vi "_f_bronkhorstWriteAuto.vi"(6 "Delay Time (s)":dbl=0.4, 8 "error in (no error)":errorcluster, 11 "Datos":T1 caption="Nuevos valores" {"Ctrl01" format="%.1f"; "Ctrl03" format="%.1f"; "Ctrl02" format="%.1f"; "Ctrl04" format="%.1f"}) -> (0 "error out":errorcluster, 1 "Dispositivos":T2=[["3", "NO", "M0000013", "Air", "1", "ln/mn", "0", "0"], ["4", "NO", "M0000014", "Air", "1", "ln/mn", "0", "0"], ["5", "NO", "M0000015", "Air", "1", "ln/mn", "0", "0"], ["6", "NO", "M0000016", "Air", "1", "ln/mn", "0", "0"], ["7", "NO", "M0000017", "Air", "1", "ln/mn", "0", "0"], ["8", "NO", "M0000018", "Air", "1", "ln/mn", "0", "0"], ["9", "NO", "M0000019", "Air", "1", "ln/mn", "0", "0"], ["10", "NO", "M0000020", "Air", "1", "ln/mn", "0", "0"], ["11", "NO", "M0000021", "Air", "1", "ln/mn", "0", "0"]] caption="MassFlowControllers")   [LabVIEW 2013]
uses:
  _f_TablaBronkhorst.ctl
  Controles/P2018 Flujos Data.ctl
  _f_BronkhorstModuleControl.ctl
  P2022 TB INCAR GLOBALES.vi
panel:
  out "Nodo":i32
  out "Dispositivos 2":string[][](table)=[["3", "NO", "M0000013", "Air", "1", "ln/mn", "0", "0"], ["4", "NO", "M0000014", "Air", "1", "ln/mn", "0", "0"], ["5", "NO", "M0000015", "Air", "1", "ln/mn", "0", "0"], ["6", "NO", "M0000016", "Air", "1", "ln/mn", "0", "0"], ["7", "NO", "M0000017", "Air", "1", "ln/mn", "0", "0"], ["8", "NO", "M0000018", "Air", "1", "ln/mn", "0", "0"], ["9", "NO", "M0000019", "Air", "1", "ln/mn", "0", "0"], ["10", "NO", "M0000020", "Air", "1", "ln/mn", "0", "0"], ["11", "NO", "M0000021", "Air", "1", "ln/mn", "0", "0"]] caption="Nuevos valores"
  out "Enable(T)":bool=TRUE
  out "VISA Bronkhorst":refnum<visa-resource-name>
  out "Num. of nodes":u32=6
  # "Cambio de setpoints automático: espere........."
  # "4"
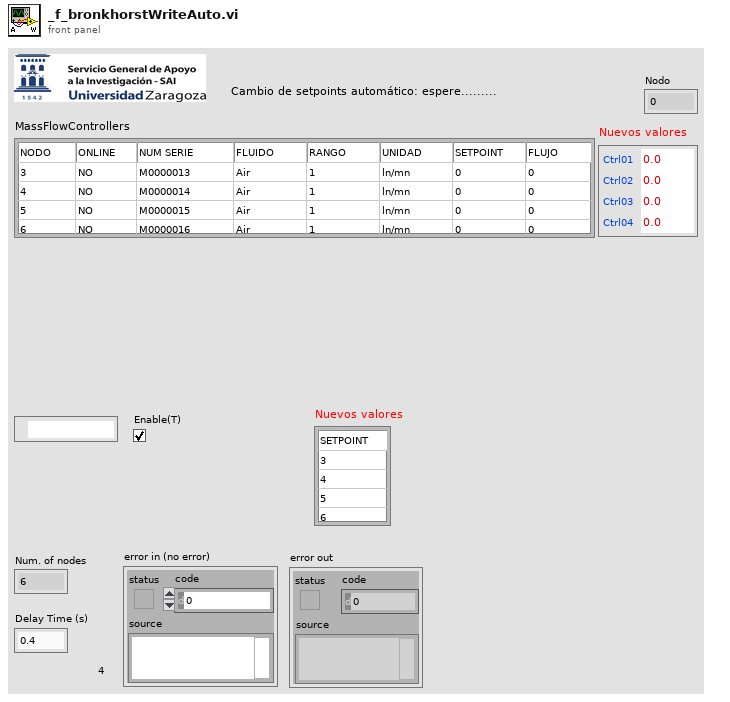
[diagram p1: front panel]
types:
  T1 = typedef "P2018 Flujos Data.ctl" = cluster{"Ctrl01":dbl, "Ctrl02":dbl, "Ctrl03":dbl, "Ctrl04":dbl}
  T2 = typedef "_f_TablaBronkhorst.ctl" = string[][]
  T3 = typedef "P2018 Bronkhorst Control.ctl" = cluster{"Dispositivos":T4, "NuevosSP":string[][], "Nodes":u32, "Delay(s)":dbl}
  T4 = typedef "_s_TablaBronkhorst.ctl" = string[][]
  T5 = typedef "P2018 Com Control.ctl" = cluster{"Flujo_1":refnum<visa-resource-name>, "Brk1":bool, "Flujo_2":refnum<visa-resource-name>, "Brk2":bool, "Flujo_3":refnum<visa-resource-name>, "Brk3":bool, "Flujo_4":refnum<visa-resource-name>, "Brk4":bool, "Eurothe":refnum<visa-resource-name>, "Eurot":bool, "Balanza":refnum<visa-resource-name>, "Bal":bool, "eValPos":refnum<visa-resource-name>, "eVal":bool, "flowbus":refnum<visa-resource-name>, "fb":bool}
  T6 = typedef "_f_BronkhorstModuleControl.ctl" = enum16{"RcharSerialNum", "RcharIdnString", "WuintFluidNum", "RuintFluidNum", "RcharFluidName", "RuintSensorType", "RfloatCap0", "RfloatCap100", "RcharCapUnitStr", "W%Setpoint", "R%Setpoint", "R%Measure", "WfloatSetpoint", "RfloatSetpoint", "RfloatMeasure ", "RfloatDensity", "WuintControlMode", "WcharRESET", "RfloatCounter", "RcharCounterUnit", "WfloatCounterLimit", "RfloatCounterLimit", "WcharCounterMode", "RcharCounterMode", "WcharCounterSPMode", "RcharCounterSPMode", "WcharCounterNewSP", "RcharCounterNewSP"}
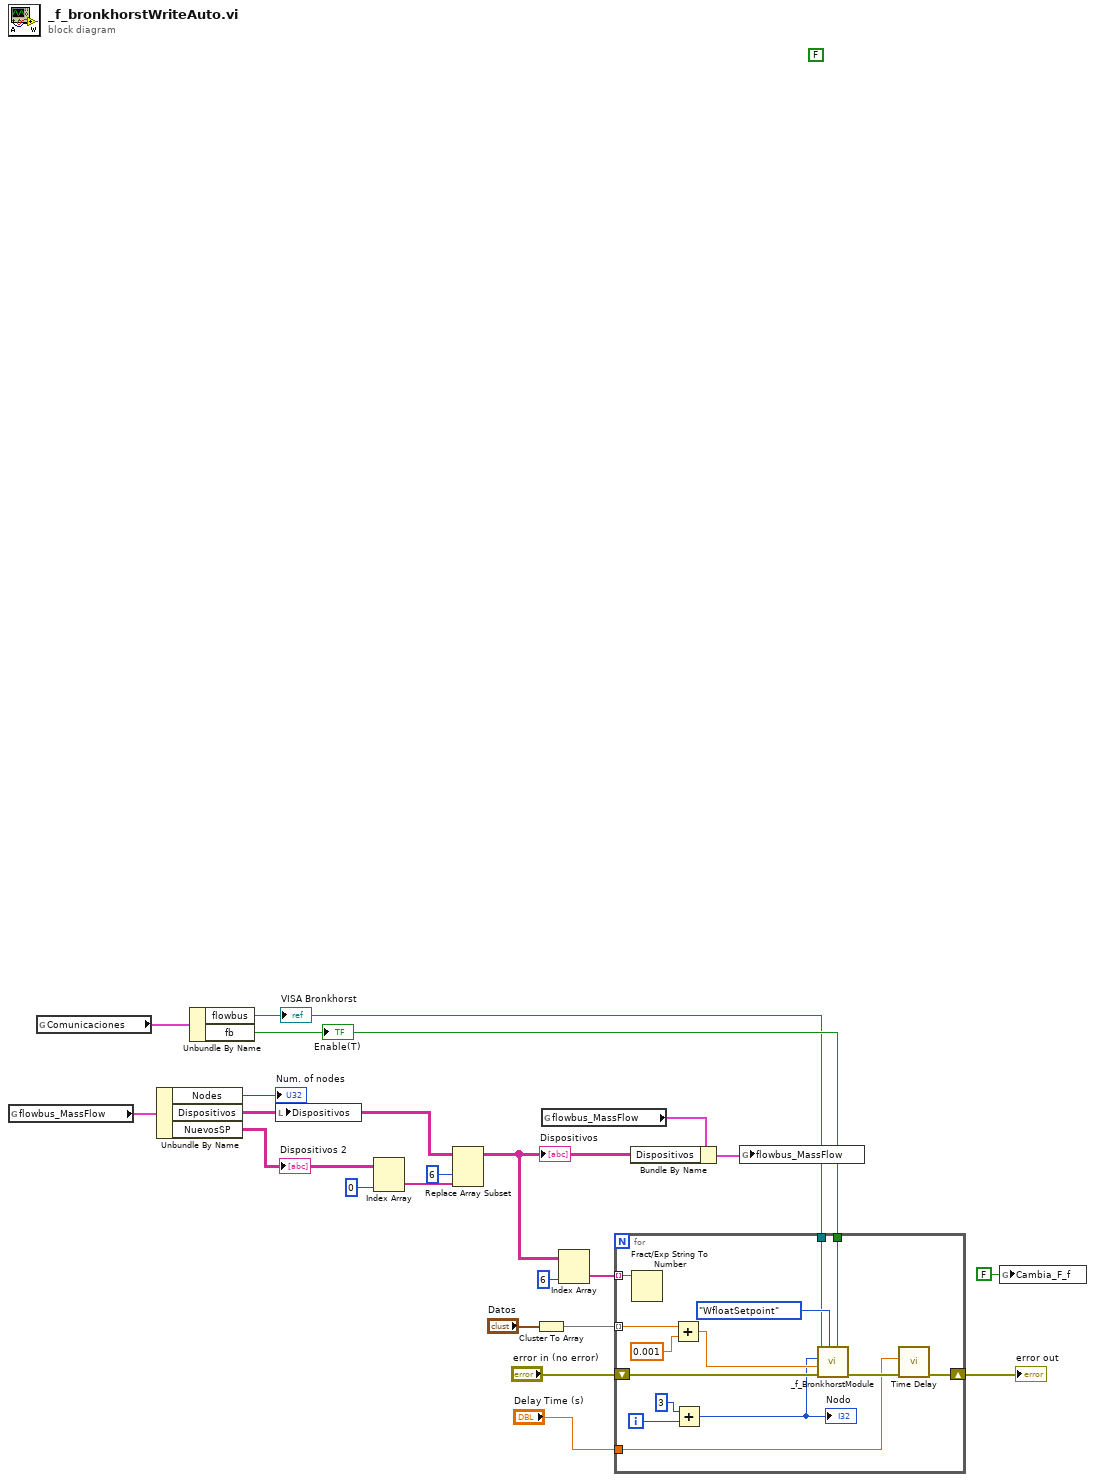
[diagram p0: block diagram]
diagram:
  (unwired) FALSE
  n1 = global read "P2022 TB INCAR GLOBALES.vi" "flowbus_MassFlow"() -> (w17:T3)
  n2 = global read "P2022 TB INCAR GLOBALES.vi" "Comunicaciones"() -> (w21:T5)
  n3 = Unbundle By Name(w17) -> ("Nodes"=→"Num. of nodes":u32, "Dispositivos"=w16:T4, "NuevosSP"=w9:string[][])
  "Dispositivos 2" <- w9
  n4 = Unbundle By Name(w21) -> ("flowbus"=w1:refnum<visa-resource-name>, "fb"=w10:bool)
  "Enable(T)" <- w10
  "VISA Bronkhorst" <- w1
  n5 = local write "Dispositivos"(w16) -> ()
  n6 = Index Array(array=w9, index (col)=0 ("disabled index (col)")) -> (element=w6:string[])  [unwired: 1 in]
  n7 = Replace Array Subset(array=w16, new element=w6, index (col)=6 ("index")) -> (w12:T4)  [unwired: 1 in]
  "Dispositivos" <- w12
  n8 = Cluster To Array(cluster="Datos") -> (array=w3:dbl[])
  n9 = global read "P2022 TB INCAR GLOBALES.vi" "flowbus_MassFlow"() -> (w20:T3)
  n10 = Index Array(array=w12, index (col)=6 ("disabled index (col)")) -> (element=w11:string[])  [unwired: 1 in]
  n11 = for {
    shift-right: [w32] -> w14
    shift-left: "error in (no error)" -> [w35]
    tunnel: w11 -> [w30] mode=indexing
    tunnel: w10 -> [w27]
    tunnel: w3 -> [w26] mode=indexing
    tunnel: "Delay Time (s)" -> [w23]
    tunnel: w1 -> [w22]
    i -> [w25]
    n12 = Fract/Exp String To Number(string=w30) -> ()  [unwired: 3 in, 2 out]
    n13 = Add(x=w26, y=0.001) -> (x+y=w29:dbl)
    n14 = Add(x=3, y=w25) -> (x+y=w24:i32)
    "Nodo" <- w24
    n15 = call "_f_BronkhorstModule.vi"("Enable(T)"=w27, "Command"=_f_BronkhorstModuleControl."WfloatSetpoint", "error in (no error)"=w35, "Value"=w29, "Nodo"=w24, "VISA resource name"=w22) -> ("error out"=w33:errorcluster)  [unwired: 2 in, 3 out]
    n16 = call "Time Delay"("error in (no error)"=w33, "Delay Time (s)"=w23) -> ("error out"=w32:errorcluster)  [unwired: 9 in]
  }
  "error out" <- w14
  n17 = Bundle By Name(cluster=w20, "Dispositivos"=w12) -> (w19:T3)
  n18 = global write "P2022 TB INCAR GLOBALES.vi" "flowbus_MassFlow"(w19) -> ()
  n19 = global write "P2022 TB INCAR GLOBALES.vi" "Cambia_F_f"(FALSE ("ChangeF")) -> ()
